vi "Problem 2.vi"() -> ()   [LabVIEW 2013, in "Problem 2.lvlib"]
uses:
  Problem 2.lvlib
panel:
  out "sum":u32
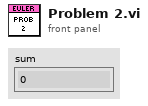
[diagram p1: front panel]
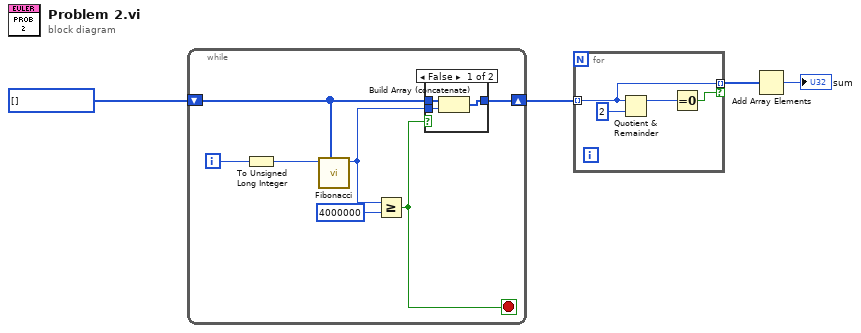
[diagram p0: block diagram]
diagram:
  n1 = while {
    shift-right: [w7] -> w3
    shift-left: u32[] [] -> [w5]
    i -> [w10]
    stop <- w6 stop-if-true
    n2 = To Unsigned Long Integer(number=w10) -> (unsigned 32bit integer=w9:u32)
    n3 = call "Fibonacci.vi"("Memo"=w5, "n"=w9) -> ("fib(n)"=w8:u32)  [unwired: 9 in]
    n4 = Greater Or Equal?(x=w8, y=u32 4000000) -> (x >= y?=w6:bool)
    n5 = case shown="False" w6 {
      tunnel: w5 -> [w14 w15]
      tunnel: w8 -> [w13 _]
      tunnel: [w12 w15] -> w7
      frame False {
        n6 = Build Array (concatenate)(w14, w13) -> (w12:u32[])
      }
      frame True {
      }
    }
  }
  n7 = for {
    tunnel: w3 -> [w18] mode=indexing
    tunnel: [w18] -> w2 mode=indexing if=w16
    n8 = Quotient & Remainder(x=w18, y=u32 2) -> (x-y*floor(x/y)=w17:u32)  [unwired: 1 out]
    n9 = Equal To 0?(x=w17) -> (x = 0?=w16:bool)
  }
  n10 = Add Array Elements(numeric array=w2) -> (sum=→"sum":u32)
